vi "Move East.vi"(11 "Map In":string[][](array[string])) -> (0 "Moved?":bool, 3 "Map Out":string[][](array[string]))   [LabVIEW 2021]
uses:
  <userlib>/_OpenG.lib/array/array.llb/Search 1D Array (String)__ogtk.vi
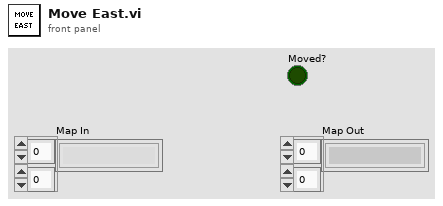
[diagram p1: front panel]
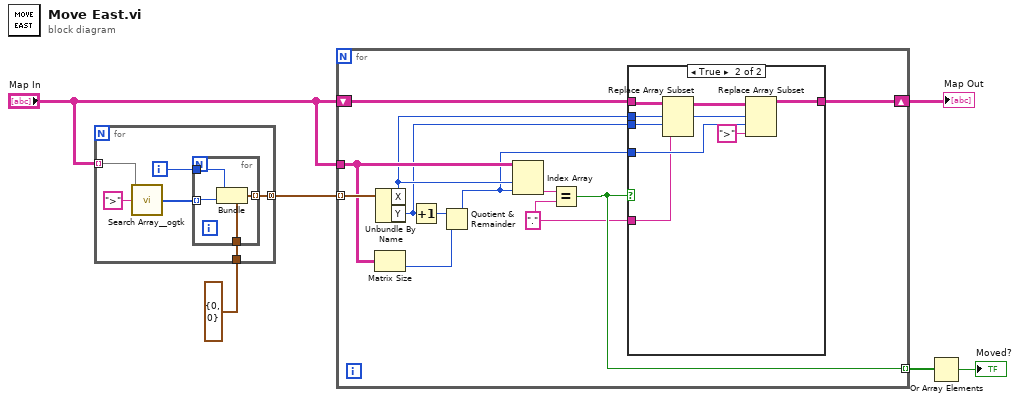
[diagram p0: block diagram]
diagram:
  n1 = for {
    tunnel: "Map In" -> [w12] mode=indexing
    tunnel: [w8] -> w5 mode=concatenating
    tunnel: cluster{"X":i32, "Y":i32} {"X"=0, "Y"=0} ("input cluster") -> [w7]
    i -> [w9]
    n2 = call-poly <userlib>:"Search Array__ogtk.vi"("Array"=w12, "Element Data"=">") -> ("Indices of Elements"=w10:i32[])  [unwired: 7 in]
    n3 = for {
      tunnel: w10 -> [w16] mode=indexing
      tunnel: w9 -> [w15]
      tunnel: [w14] -> w8 mode=indexing
      tunnel: w7 -> [w13]
      n4 = Bundle(cluster=w13, "X"=w15, "Y"=w16) -> (w14:cluster{"X":i32, "Y":i32})
    }
  }
  n5 = for {
    shift-right: [w22] -> w1
    shift-left: "Map In" -> [w23]
    tunnel: "Map In" -> [w26]
    tunnel: w5 -> [w28] mode=indexing
    tunnel: [w21] -> w3 mode=indexing
    w17 = "."
    n6 = Matrix Size(0:w26) -> (2:w25:i32)  [unwired: 1 out]
    n7 = Unbundle By Name(w28) -> ("X"=w20:i32, "Y"=w19:i32)
    n8 = Increment(x=w19) -> (x+1=w27:i32)
    n9 = Quotient & Remainder(x=w27, y=w25) -> (x-y*floor(x/y)=w18:i32)  [unwired: 1 out]
    n10 = Index Array(array=w26, index (row)=w20, index (col)=w18) -> (element=w24:string)
    n11 = Equal?(x=w24, y=w17) -> (x = y?=w21:bool)
    n12 = case shown="True" w21 {
      tunnel: w23 -> [w29 w37]
      tunnel: [w29 w35] -> w22
      tunnel: w20 -> [_ w34]
      tunnel: w19 -> [_ w33]
      tunnel: w18 -> [_ w32]
      tunnel: w17 -> [_ w31]
      frame False {
      }
      frame True {
        n13 = Replace Array Subset(array=w37, new element=w31, index (row)=w34, index (col)=w33) -> (w36:string[][])
        n14 = Replace Array Subset(array=w36, new element=">" ("new element/subarray"), index (row)=w34, index (col)=w32) -> (w35:string[][])
      }
    }
  }
  "Map Out" <- w1
  n15 = Or Array Elements(Boolean array=w3) -> (logical OR=→"Moved?":bool)
